vi "SR830-value-to-str(SubVI).vi"(8 "电流":dbl format="%#_13g", 11 "Parameter Values":T1) -> (3 "数组":string[](array[string]))   [LabVIEW 2019, in "SubVI.lvlib"]
uses:
  SubVI.lvlib
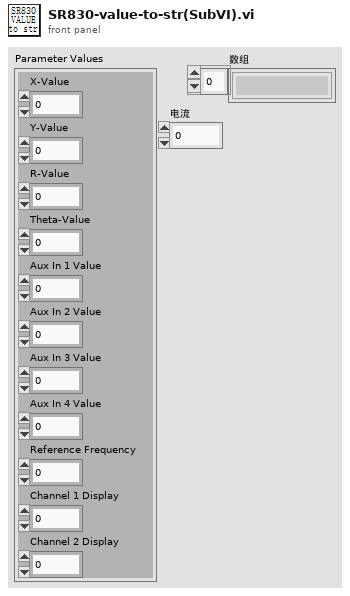
[diagram p1: front panel]
types:
  T1 = cluster{"X-Value":dbl, "Y-Value":dbl, "R-Value":dbl, "Theta-Value":dbl, "Aux In 1 Value":dbl, "Aux In 2 Value":dbl, "Aux In 3 Value":dbl, "Aux In 4 Value":dbl, "Reference Frequency":dbl, "Channel 1 Display":dbl, "Channel 2 Display":dbl}
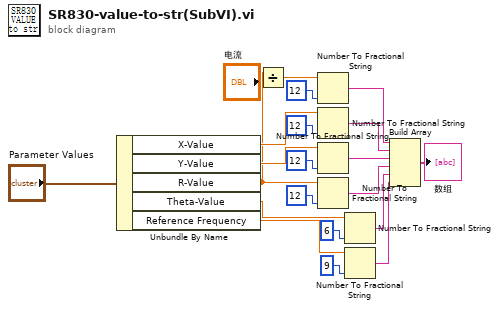
[diagram p0: block diagram]
diagram:
  n1 = Unbundle By Name("Parameter Values") -> ("X-Value"=w7:dbl, "Y-Value"=w10:dbl, "R-Value"=w5:dbl, "Theta-Value"=w17:dbl, "Reference Frequency"=w20:dbl)
  n2 = Divide(x=w5, y="电流") -> (x/y=w3:dbl)
  n3 = Number To Fractional String(number=w3, precision (6)=i16 12 ("精度(6)")) -> (F-format string=w1:string)  [unwired: 2 in]
  n4 = Number To Fractional String(number=w7, precision (6)=i16 12 ("精度(6)")) -> (F-format string=w14:string)  [unwired: 2 in]
  n5 = Number To Fractional String(number=w10, precision (6)=i16 12 ("精度(6)")) -> (F-format string=w15:string)  [unwired: 2 in]
  n6 = Number To Fractional String(number=w5, precision (6)=i16 12 ("精度(6)")) -> (F-format string=w16:string)  [unwired: 2 in]
  n7 = Number To Fractional String(number=w17, precision (6)=i16 6 ("精度(6)")) -> (F-format string=w18:string)  [unwired: 2 in]
  n8 = Number To Fractional String(number=w20, precision (6)=i16 9 ("精度(6)")) -> (F-format string=w19:string)  [unwired: 2 in]
  n9 = Build Array(w1, w14, w15, w16, w18, w19) -> (→"数组":string[])
